vi "4.1.vi"(8 "error in (no error)":errorcluster, 9 "Min Temp":dbl, 10 "Max Temp":dbl, 11 "Current Temp":dbl) -> (0 "error out":errorcluster, 1 "Warning Y/N":bool, 2 "Warning Text":string)   [LabVIEW 2014]
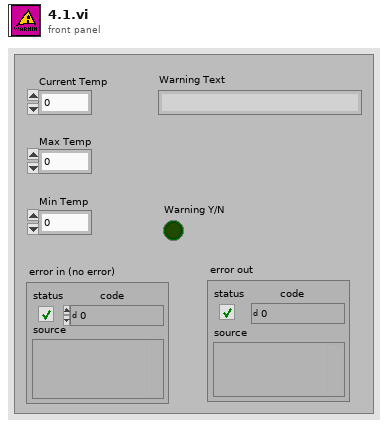
[diagram p1: front panel]
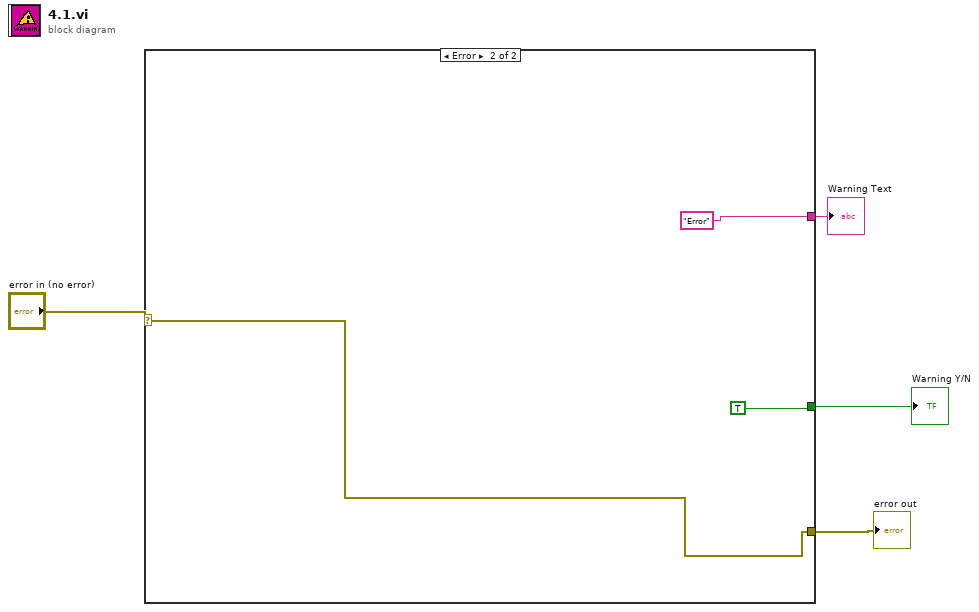
[diagram p0: block diagram]
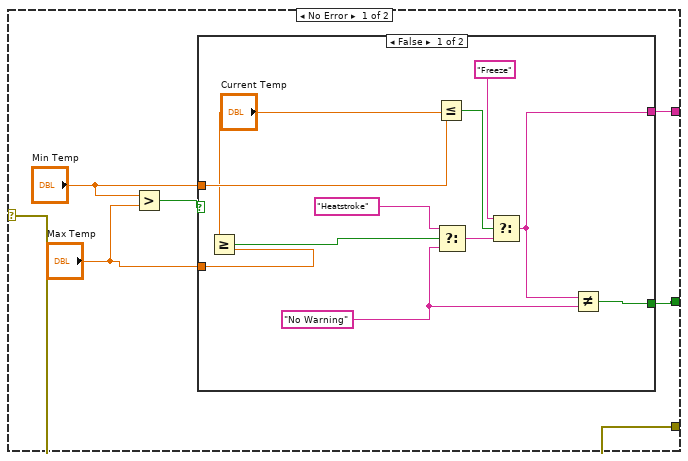
[diagram p2: hidden frame]
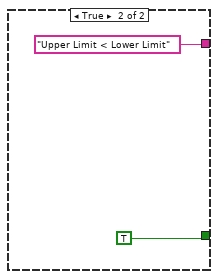
[diagram p3: hidden frame]
diagram:
  n1 = case shown="Error" "error in (no error)" {
    selector: "error in (no error)" -> [w5 w26]
    tunnel: [w10 "Error"] -> w4
    tunnel: [w9 TRUE] -> w3
    tunnel: [w5 w26] -> w1
    frame No Error {
      n2 = Greater?(x="Min Temp", y="Max Temp") -> (0:w7:bool)
      n3 = case shown="False" w7 {
        tunnel: [w17 "Upper Limit < Lower Limit"] -> w10
        tunnel: [w11 TRUE] -> w9
        tunnel: "Max Temp" -> [w14 _]
        tunnel: "Min Temp" -> [w13 _]
        frame False {
          w16 = "No Warning"
          n4 = Greater Or Equal?(x="Current Temp", y=w14) -> (x >= y?=w15:bool)
          n5 = Less Or Equal?(x="Current Temp", y=w13) -> (x <= y?=w21:bool)
          n6 = Select(t="Heatstroke", s=w15, f=w16) -> (s? t:f=w18:string)
          n7 = Select(t="Freeze", s=w21, f=w18) -> (s? t:f=w17:string)
          n8 = Not Equal?(x=w17, y=w16) -> (x != y?=w11:bool)
        }
        frame True {
        }
      }
    }
    frame Error {
    }
  }
  "Warning Text" <- w4
  "Warning Y/N" <- w3
  "error out" <- w1
